vi "2.0.0_Firware Version Check.vi"(6 ".batCM":T1={"Brush_ADC.bat"="Brush_ADC.bat", "Get Release Version.bat"="Get Release Version.bat", "Getting Software  Version.bat"="Getting Software  Version.bat", "Pump_ADC.bat"="Pump_ADC.bat", "Starting  Pump Motor.bat"="Starting  Pump Motor.bat", "Starting  Test Mode.bat"="Starting  Test Mode.bat", "Starting Brush Motor 1.bat"="Starting Brush Motor 1.bat", "Starting Brush Motor 2.bat"="Starting Brush Motor 2.bat", "Starting Brush Motor 3.bat"="Starting Brush Motor 3.bat", "Starting LED Test.bat"="Starting LED Test.bat", "Stopping  Brush Motor.bat"="Stopping  Brush Motor.bat", "Stopping  Pump Motor.bat"="Stopping  Pump Motor.bat", "Stopping  Test Mode.bat"="Stopping  Test Mode.bat", "Starting Self Test.bat"="Starting Self Test.bat", "Software Reset.bat"="Software Reset.bat", "Get HW version.bat"="Get HW version.bat", "Read PMIC status.bat"="Read PMIC status.bat", "SC IMU Data Streaming.bat"="SC IMU Data Streaming.bat"}, 7 "Data in":T2, 8 "error in (no error)":errorcluster, 9 "AllControls In":T3, 10 "?":T4, 11 "Message Queue out":T5) -> (0 "error out":errorcluster, 1 "Flow":string, 2 "Data":T4, 3 "Message Queue Out":T5, 5 "Data out":T2)   [LabVIEW 2017]
uses:
  Depends/AMC/subVIs/TypeDefs/amc_Message Queue.ctl
  Depends/AMC/subVIs/TypeDefs/amc_Message.ctl
  Depends/Tools/Keyed Array/Tools_KeyedArray KeyedArray.ctl
  Ctrls/Data.ctl
  Ctrls/AllControls.ctl
  Ctrls/CSV_Data.ctl
  0516/X682 Chassis Connectivity Tester Program/Ctrls/682_cmd.ctl
types:
  T1 = typedef "682_cmd.ctl" = cluster{"Brush_ADC.bat":string, "Get Release Version.bat":string, "Getting Software  Version.bat":string, "Pump_ADC.bat":string, "Starting  Pump Motor.bat":string, "Starting  Test Mode.bat":string, "Starting Brush Motor 1.bat":string, "Starting Brush Motor 2.bat":string, "Starting Brush Motor 3.bat":string, "Starting LED Test.bat":string, "Stopping  Brush Motor.bat":string, "Stopping  Pump Motor.bat":string, "Stopping  Test Mode.bat":string, "Starting Self Test.bat":string, "Software Reset.bat":string, "Get HW version.bat":string, "Read PMIC status.bat":string, "SC IMU Data Streaming.bat":string}
  T2 = typedef "CSV_Data.ctl" = cluster{"Initialisation":cluster{"LMT - Connect UUT (con COM)":string, "LMT - Software Version (rrel)":string, "LMT - Write SKU file (wskuc)":string, "LMT - SKU file name":string, "Connect UUT DDM":string, "Read DDM EOL Timestamp - Mode":string, "Read DDM EOL Timestamp - Timestamp":string, "Read DDM EOL Timestamp - Rig ID":string, "Read DDM EOL Timestamp - Passmark ID":string, "Read DDM EOL Timestamp - Passmark Rev":string, "Software Version before flashing":string, "Read Hardware Serial":string, "UUT DDM SN":string, "Compare DDM SN with MES SN":string, "Backup PCBA Calibration EEPROM Response - CAL":string, "Flash Firmware Version":string, "Check SW Version":string, "Read DDM SW Version after flashing":string, "Set SKU Config":string, "Ready Status":string, "Set Device Mode to EOL":string, "DDM Parameter - Voltage":string, "DDM Parameter - Current":string, "DDM Parameter - Power":string, "DDM Parameter - Speed":string, "DDM Parameter - Pressure":string, "Tester Parameter - Voltage":string, "Tester Parameter - Current":string, "Tester Parameter - Power":string, "Tester Parameter - Ambient Pressure":string, "Tester Parameter - Ambient Temperature":string, "Calculated Parameter - DDM Pressure Corrected":string, "Calculated Parameter - DDM Real Power":string, "Calculated Parameter - Delta V":string}, "BEMF_Calibration":cluster{"Calibration Result - eol_cold_bemf_temp":string, "DDM Ambient Temp":string, "Restriction Plate Diameter":string, "Calibration Result - eol_bemf_mp_cold_coef_a":string, "Calibration Result - eol_bemf_mp_cold_coef_b":string, "Calibration Result - eol_bemf_mp_cold_coef_c":string, "Calibration Result - eol_bemf_lsi_cold_ref_coeffs":string, "Get - Calibration Result - eol_bemf_lsi_speed":string, "Get - Calibration Result - eol_bemf_lsi_integral_0":string, "Calibration Result - eol_bemf_lsi_integral_1":string, "Get - Calibration Result - eol_bemf_lsi_integral_2":string, "Get - Calibration Result - eol_cold_bemf":string, "Get - Calibration Result - eol_cold_bemf_fisf":string, "Finalise Calibration":string, "Compare -Calibration Result - eol_cold_bemf":string, "Compare -Calibration Result - eol_cold_bemf_fisf":string}, "ECO":cluster{"Reset Power Tune":string, "Reset BEMF FISF Calibration":string, "Restriction Plate Diameter":string, "ECO - Stabilisation Time":string, "ECO - DDM Parameter - Voltage":string, "ECO - DDM Parameter - Current":string, "ECO - DDM Parameter - Power":string, "ECO - DDM Parameter - Measured Power":string, "ECO - DDM Parameter - Speed":string, "ECO - DDM Parameter - Pressure":string, "ECO - Tester Parameter - Voltage":string, "ECO - Tester Parameter - Current":string, "ECO - Tester Parameter - Power":string, "ECO - Tester Parameter - Ambient Pressure":string, "ECO - Tester Parameter - Ambient Temperature":string, "ECO - Tester Parameter - Ambient Humidity":string, "ECO - Calculated Parameter - DDM Pressure Corrected":string, "ECO - Calculated Parameter - DDM Real Power":string, "ECO - Calculated Parameter - Delta V":string, "ECO - Calculated Parameter - Flowrate":string, "ECO - Calculated Parameter - Airwatt":string, "ECO - Formula":string, "PT ECO - Power Tune Mode Status":string}, "BOOST":cluster{"Restriction Plate Diameter":string, "BOOST - Stabilisation Time":string, "BOOST - DDM Parameter - Voltage":string, "BOOST - DDM Parameter - Current":string, "BOOST - DDM Parameter - Power":string, "BOOST - DDM Parameter - Measured Power":string, "BOOST - DDM Parameter - Speed":string, "BOOST - DDM Parameter - Pressure":string, "BOOST - Tester Parameter - Voltage":string, "BOOST - Tester Parameter - Current":string, "BOOST - Tester Parameter - Power":string, "BOOST - Tester Parameter - Ambient Pressure":string, "BOOST - Tester Parameter - Ambient Temperature":string, "BOOST - Tester Parameter - Ambient Humidity":string, "BOOST - Calculated Parameter - DDM Pressure Corrected":string, "BOOST - Calculated Parameter - DDM Real Power":string, "BOOST - Calculated Parameter - Delta V":string, "BOOST - Calculated Parameter - Flowrate":string, "BOOST - Calculated Parameter - Airwatt":string, "BOOST - Get AM Presence":string, "Air Muscle Turn Off Status":string, "BOOST - Air Muscle Calculated Parameter - Airwatt B":string, "BOOST - Air Muscle Calculate Airwatt Delta":string, "PT BOOST - Power Tune Mode Status":string, "Finalise Calibration":string, "ECO - Get AW Calibration value":string, "BOOST - Get AW Calibration value":string}, "MAX":cluster{"Restriction Plate Diameter":string, "MAX - Stabilisation Time":string, "Get Average Delta Tmag (LSIdelta_FISFdelta_LSItmag_FISFtmag_IIRtmag)":string, "Get Average Delta Tmag FISF":string, "MAX - DDM Parameter - Voltage":string, "MAX - DDM Parameter - Current":string, "MAX - DDM Parameter - Power":string, "MAX - DDM Parameter - Measured Power":string, "MAX - DDM Parameter - Speed":string, "MAX - DDM Parameter - Pressure":string, "MAX - Tester Parameter - Voltage":string, "MAX - Tester Parameter - Current":string, "MAX - Tester Parameter - Power":string, "MAX - Tester Parameter - Ambient Pressure":string, "MAX - Tester Parameter - Ambient Temperature":string, "MAX - Tester Parameter - Ambient Humidity":string, "MAX - Calculated Parameter - DDM Pressure Corrected":string, "MAX - Calculated Parameter - DDM Real Power":string, "MAX - Calculated Parameter - Delta V":string, "MAX - Calculated Parameter - Flowrate":string, "MAX - Calculated Parameter - Airwatt":string, "MAX_FISF_Check_Average_Delta_Tmag":string, "MAX - FISF - BEMF Finetune Result":string, "MAX tune - Delta P1":string, "MAX tune - Calculated Parameter - Airwatt":string, "Calculate Delta Airwatts - MAX finetune - Delta P2":string, "MAX finetune - DDM Parameter - Voltage":string, "MAX finetune - DDM Parameter - Current":string, "MAX finetune - DDM Parameter - Power":string, "MAX finetune - DDM Parameter - Measured Power":string, "MAX finetune - DDM Parameter - Speed":string, "MAX finetune - DDM Parameter - Pressure":string, "MAX finetune - Tester Parameter - Voltage":string, "MAX finetune - Tester Parameter - Current":string, "MAX finetune - Tester Parameter - Power":string, "MAX finetune - Tester Parameter - Ambient Pressure":string, "MAX finetune - Tester Parameter - Ambient Temperature":string, "MAX finetune - Tester Parameter - Ambient Humidity":string, "MAX finetune - Calculated Parameter - DDM Pressure Corrected":string, "MAX finetune - Calculated Parameter - DDM Real Power":string, "MAX finetune - Calculated Parameter - Delta V":string, "MAX finetune - Calculated Parameter - Flowrate":string, "MAX finetune - Calculated Parameter - Airwatt":string, "Check Derate Result":string, "Delta Tmag FISF":string, "Get Hot BEMF Result":string, "Calculate delta Pressure":string, "Finalise Calibration":string, "Calculate & Check Delta BEMF":string, "Delta P Airwatts Value":string}, "LL":cluster{"DDM Ambient Temp":string, "Restriction Plate Diameter":string, "LL - DDM Parameter - Voltage":string, "LL - DDM Parameter - Current":string, "LL - DDM Parameter - Power":string, "LL - DDM Parameter - Measured Power":string, "LL - DDM Parameter - Speed":string, "LL - DDM Parameter - Pressure":string, "LL - Tester Parameter - Voltage":string, "LL - Tester Parameter - Current":string, "LL - Tester Parameter - Power":string, "LL - DDM Real Power":string, "LL - Calibrate Task Detect LL":string}, "HL":cluster{"HL - DDM Parameter - Voltage":string, "HL - DDM Parameter - Current":string, "HL - DDM Parameter - Power":string, "HL - DDM Parameter - Measured Power":string, "HL - DDM Parameter - Speed":string, "HL - DDM Parameter - Pressure":string, "HL - Tester Parameter - Voltage":string, "HL - Tester Parameter - Current":string, "HL - Tester Parameter - Power":string, "HL - DDM Real Power":string, "HL - Calibrate Task Detect HL":string}, "LH":cluster{"Restriction Plate Diameter":string, "LH - DDM Parameter - Voltage":string, "LH - DDM Parameter - Current":string, "LH - DDM Parameter - Power":string, "LH - DDM Parameter - Measured Power":string, "LH - DDM Parameter - Speed":string, "LH - DDM Parameter - Pressure":string, "LH - Tester Parameter - Voltage":string, "LH - Tester Parameter - Current":string, "LH - Tester Parameter - Power":string, "LH - DDM Real Power":string, "LH - Calibrate Task Detect LH":string}, "HH":cluster{"HH - DDM Parameter - Voltage":string, "HH - DDM Parameter - Current":string, "HH - DDM Parameter - Power":string, "HH - DDM Parameter - Measured Power":string, "HH - DDM Parameter - Speed":string, "HH - DDM Parameter - Pressure":string, "HH - Tester Parameter - Voltage":string, "HH - Tester Parameter - Current":string, "HH - Tester Parameter - Power":string, "HH - DDM Real Power":string, "HH - Calibrate Task Detect HH":string}, "Inlet Blockage Calibration":cluster{"Inlet Blockage Calibration - DDM Parameter - Voltage":string, "Inlet Blockage Calibration - DDM Parameter - Current":string, "Inlet Blockage Calibration - DDM Parameter - Power":string, "Inlet Blockage Calibration - DDM Parameter - Measured Power":string, "Inlet Blockage Calibration - DDM Parameter - Speed":string, "Inlet Blockage Calibration - DDM Parameter - Pressure":string, "Inlet Blockage Calibration - Tester Parameter - Voltage":string, "Inlet Blockage Calibration - Tester Parameter - Current":string, "Inlet Blockage Calibration - Tester Parameter - Power":string, "Inlet Blockage Calibration - DDM Real Power":string, "Calibration Inlet Blockage_E":string, "Finalise Calibration":string, "Get Task Detect LL":string, "Get Task Detect HL":string, "Get Task Detect LH":string, "Get Task Detect HH":string, "Calibration Inlet Blockage":string, "Calibration eol cold bemf temp":string}, "GOOD":cluster{"GOOD UNIT - Clear EEPROM Error Log":string, "GOOD UNIT - Write Product Timestamp - Mode":string, "GOOD UNIT - Write Product Timestamp - Timestamp":string, "GOOD UNIT - Write Product Timestamp - Rig ID":string, "GOOD UNIT - Write Product Timestamp - Passmark ID":string, "GOOD UNIT - Write Product Timestamp - Passmark Rev":string, "GOOD UNIT - Set Device Mode to PROD":string, "GOOD UNIT - Backup PCBA Calibration EEPROM Response":string, "GOOD UNIT - Check Security Bit":string, "GOOD UNIT - Set Calibration Lock":string, "GOOD UNIT - Get_Calibration_Lock":string, "GOOD UNIT - Disconnect UUT":string}, "NG":cluster{"NG UNIT - Read NVM Error":string, "NG UNIT - Set Device Mode to FCT":string, "NG UNIT - Backup PCBA Calibration EEPROM Response - CAL":string, "NG UNIT - Backup PCBA Calibration EEPROM Response - ERROR":string, "NG UNIT - Backup PCBA Calibration EEPROM Response - USAGE":string, "NG UNIT - Disconnect UUT":string}, "SN":string, "Table":string[][], "Count":cluster{"Total":i32, "OK":i32, "NG":i32, "Yield":dbl}, "Start Time":timestamp, "daemon reference":refnum<k5>, "CT":dbl, "Config":string[][], "OK/NG":bool, "Station ID":string, "MES DDM SN":string, "MES PCBA SN":string, "Retest":string, "Lux":string, "Initialisation_Status":cluster{"LMT - Connect UUT (con COM)":string, "LMT - Software Version (rrel)":string, "LMT - Write SKU file (wskuc)":string, "LMT - SKU file name":string, "Connect UUT DDM":string, "Read DDM EOL Timestamp - Mode":string, "Read DDM EOL Timestamp - Timestamp":string, "Read DDM EOL Timestamp - Rig ID":string, "Read DDM EOL Timestamp - Passmark ID":string, "Read DDM EOL Timestamp - Passmark Rev":string, "Software Version before flashing":string, "Read Hardware Serial":string, "UUT DDM SN":string, "Compare DDM SN with MES SN":string, "Backup PCBA Calibration EEPROM Response - CAL":string, "Flash Firmware Version":string, "Check SW Version":string, "Read DDM SW Version after flashing":string, "Set SKU Config":string, "Ready Status":string, "Set Device Mode to EOL":string, "DDM Parameter - Voltage":string, "DDM Parameter - Current":string, "DDM Parameter - Power":string, "DDM Parameter - Speed":string, "DDM Parameter - Pressure":string, "Tester Parameter - Voltage":string, "Tester Parameter - Current":string, "Tester Parameter - Power":string, "Tester Parameter - Ambient Pressure":string, "Tester Parameter - Ambient Temperature":string, "Calculated Parameter - DDM Pressure Corrected":string, "Calculated Parameter - DDM Real Power":string, "Calculated Parameter - Delta V":string}, "BEMF_Calibration_Status":cluster{"Calibration Result - eol_cold_bemf_temp":string, "DDM Ambient Temp":string, "Restriction Plate Diameter":string, "Calibration Result - eol_bemf_mp_cold_coef_a":string, "Calibration Result - eol_bemf_mp_cold_coef_b":string, "Calibration Result - eol_bemf_mp_cold_coef_c":string, "Calibration Result - eol_bemf_lsi_cold_ref_coeffs":string, "Get - Calibration Result - eol_bemf_lsi_speed":string, "Get - Calibration Result - eol_bemf_lsi_integral_0":string, "Calibration Result - eol_bemf_lsi_integral_1":string, "Get - Calibration Result - eol_bemf_lsi_integral_2":string, "Get - Calibration Result - eol_cold_bemf":string, "Get - Calibration Result - eol_cold_bemf_fisf":string, "Finalise Calibration":string, "Compare -Calibration Result - eol_cold_bemf":string, "Compare -Calibration Result - eol_cold_bemf_fisf":string}, "ECO_Status":cluster{"Reset Power Tune":string, "Reset BEMF FISF Calibration":string, "Restriction Plate Diameter":string, "ECO - Stabilisation Time":string, "ECO - DDM Parameter - Voltage":string, "ECO - DDM Parameter - Current":string, "ECO - DDM Parameter - Power":string, "ECO - DDM Parameter - Measured Power":string, "ECO - DDM Parameter - Speed":string, "ECO - DDM Parameter - Pressure":string, "ECO - Tester Parameter - Voltage":string, "ECO - Tester Parameter - Current":string, "ECO - Tester Parameter - Power":string, "ECO - Tester Parameter - Ambient Pressure":string, "ECO - Tester Parameter - Ambient Temperature":string, "ECO - Tester Parameter - Ambient Humidity":string, "ECO - Calculated Parameter - DDM Pressure Corrected":string, "ECO - Calculated Parameter - DDM Real Power":string, "ECO - Calculated Parameter - Delta V":string, "ECO - Calculated Parameter - Flowrate":string, "ECO - Calculated Parameter - Airwatt":string, "ECO - Formula":string, "PT ECO - Power Tune Mode Status":string}, "BOOST_Status":cluster{"Restriction Plate Diameter":string, "BOOST - Stabilisation Time":string, "BOOST - DDM Parameter - Voltage":string, "BOOST - DDM Parameter - Current":string, "BOOST - DDM Parameter - Power":string, "BOOST - DDM Parameter - Measured Power":string, "BOOST - DDM Parameter - Speed":string, "BOOST - DDM Parameter - Pressure":string, "BOOST - Tester Parameter - Voltage":string, "BOOST - Tester Parameter - Current":string, "BOOST - Tester Parameter - Power":string, "BOOST - Tester Parameter - Ambient Pressure":string, "BOOST - Tester Parameter - Ambient Temperature":string, "BOOST - Tester Parameter - Ambient Humidity":string, "BOOST - Calculated Parameter - DDM Pressure Corrected":string, "BOOST - Calculated Parameter - DDM Real Power":string, "BOOST - Calculated Parameter - Delta V":string, "BOOST - Calculated Parameter - Flowrate":string, "BOOST - Calculated Parameter - Airwatt":string, "BOOST - Get AM Presence":string, "Air Muscle Turn Off Status":string, "BOOST - Air Muscle Calculated Parameter - Airwatt B":string, "BOOST - Air Muscle Calculate Airwatt Delta":string, "PT BOOST - Power Tune Mode Status":string, "Finalise Calibration":string, "ECO - Get AW Calibration value":string, "BOOST - Get AW Calibration value":string}, "MAX_Status":cluster{"Restriction Plate Diameter":string, "MAX - Stabilisation Time":string, "Get Average Delta Tmag (LSIdelta_FISFdelta_LSItmag_FISFtmag_IIRtmag)":string, "Get Average Delta Tmag FISF":string, "MAX - DDM Parameter - Voltage":string, "MAX - DDM Parameter - Current":string, "MAX - DDM Parameter - Power":string, "MAX - DDM Parameter - Measured Power":string, "MAX - DDM Parameter - Speed":string, "MAX - DDM Parameter - Pressure":string, "MAX - Tester Parameter - Voltage":string, "MAX - Tester Parameter - Current":string, "MAX - Tester Parameter - Power":string, "MAX - Tester Parameter - Ambient Pressure":string, "MAX - Tester Parameter - Ambient Temperature":string, "MAX - Tester Parameter - Ambient Humidity":string, "MAX - Calculated Parameter - DDM Pressure Corrected":string, "MAX - Calculated Parameter - DDM Real Power":string, "MAX - Calculated Parameter - Delta V":string, "MAX - Calculated Parameter - Flowrate":string, "MAX - Calculated Parameter - Airwatt":string, "MAX_FISF_Check_Average_Delta_Tmag":string, "MAX - FISF - BEMF Finetune Result":string, "MAX tune - Delta P1":string, "MAX tune - Calculated Parameter - Airwatt":string, "Calculate Delta Airwatts - MAX finetune - Delta P2":string, "MAX finetune - DDM Parameter - Voltage":string, "MAX finetune - DDM Parameter - Current":string, "MAX finetune - DDM Parameter - Power":string, "MAX finetune - DDM Parameter - Measured Power":string, "MAX finetune - DDM Parameter - Speed":string, "MAX finetune - DDM Parameter - Pressure":string, "MAX finetune - Tester Parameter - Voltage":string, "MAX finetune - Tester Parameter - Current":string, "MAX finetune - Tester Parameter - Power":string, "MAX finetune - Tester Parameter - Ambient Pressure":string, "MAX finetune - Tester Parameter - Ambient Temperature":string, "MAX finetune - Tester Parameter - Ambient Humidity":string, "MAX finetune - Calculated Parameter - DDM Pressure Corrected":string, "MAX finetune - Calculated Parameter - DDM Real Power":string, "MAX finetune - Calculated Parameter - Delta V":string, "MAX finetune - Calculated Parameter - Flowrate":string, "MAX finetune - Calculated Parameter - Airwatt":string, "Check Derate Result":string, "Delta Tmag FISF":string, "Get Hot BEMF Result":string, "Calculate delta Pressure":string, "Finalise Calibration":string, "Calculate & Check Delta BEMF":string, "Delta P Airwatts Value":string}, "LL_Status":cluster{"DDM Ambient Temp":string, "Restriction Plate Diameter":string, "LL - DDM Parameter - Voltage":string, "LL - DDM Parameter - Current":string, "LL - DDM Parameter - Power":string, "LL - DDM Parameter - Measured Power":string, "LL - DDM Parameter - Speed":string, "LL - DDM Parameter - Pressure":string, "LL - Tester Parameter - Voltage":string, "LL - Tester Parameter - Current":string, "LL - Tester Parameter - Power":string, "LL - DDM Real Power":string, "LL - Calibrate Task Detect LL":string}, "HL_Status":cluster{"HL - DDM Parameter - Voltage":string, "HL - DDM Parameter - Current":string, "HL - DDM Parameter - Power":string, "HL - DDM Parameter - Measured Power":string, "HL - DDM Parameter - Speed":string, "HL - DDM Parameter - Pressure":string, "HL - Tester Parameter - Voltage":string, "HL - Tester Parameter - Current":string, "HL - Tester Parameter - Power":string, "HL - DDM Real Power":string, "HL - Calibrate Task Detect HL":string}, "LH_Status":cluster{"Restriction Plate Diameter":string, "LH - DDM Parameter - Voltage":string, "LH - DDM Parameter - Current":string, "LH - DDM Parameter - Power":string, "LH - DDM Parameter - Measured Power":string, "LH - DDM Parameter - Speed":string, "LH - DDM Parameter - Pressure":string, "LH - Tester Parameter - Voltage":string, "LH - Tester Parameter - Current":string, "LH - Tester Parameter - Power":string, "LH - DDM Real Power":string, "LH - Calibrate Task Detect LH":string}, "HH_Status":cluster{"HH - DDM Parameter - Voltage":string, "HH - DDM Parameter - Current":string, "HH - DDM Parameter - Power":string, "HH - DDM Parameter - Measured Power":string, "HH - DDM Parameter - Speed":string, "HH - DDM Parameter - Pressure":string, "HH - Tester Parameter - Voltage":string, "HH - Tester Parameter - Current":string, "HH - Tester Parameter - Power":string, "HH - DDM Real Power":string, "HH - Calibrate Task Detect HH":string}, "Inlet Blockage Calibration_Status":cluster{"Inlet Blockage Calibration - DDM Parameter - Voltage":string, "Inlet Blockage Calibration - DDM Parameter - Current":string, "Inlet Blockage Calibration - DDM Parameter - Power":string, "Inlet Blockage Calibration - DDM Parameter - Measured Power":string, "Inlet Blockage Calibration - DDM Parameter - Speed":string, "Inlet Blockage Calibration - DDM Parameter - Pressure":string, "Inlet Blockage Calibration - Tester Parameter - Voltage":string, "Inlet Blockage Calibration - Tester Parameter - Current":string, "Inlet Blockage Calibration - Tester Parameter - Power":string, "Inlet Blockage Calibration - DDM Real Power":string, "Calibration Inlet Blockage_E":string, "Finalise Calibration":string, "Get Task Detect LL":string, "Get Task Detect HL":string, "Get Task Detect LH":string, "Get Task Detect HH":string, "Calibration Inlet Blockage":string, "Calibration eol cold bemf temp":string}, "GOOD_Status":cluster{"GOOD UNIT - Clear EEPROM Error Log":string, "GOOD UNIT - Write Product Timestamp - Mode":string, "GOOD UNIT - Write Product Timestamp - Timestamp":string, "GOOD UNIT - Write Product Timestamp - Rig ID":string, "GOOD UNIT - Write Product Timestamp - Passmark ID":string, "GOOD UNIT - Write Product Timestamp - Passmark Rev":string, "GOOD UNIT - Set Device Mode to PROD":string, "GOOD UNIT - Backup PCBA Calibration EEPROM Response":string, "GOOD UNIT - Check Security Bit":string, "GOOD UNIT - Set Calibration Lock":string, "GOOD UNIT - Get_Calibration_Lock":string, "GOOD UNIT - Disconnect UUT":string}, "NG_Status":cluster{"NG UNIT - Read NVM Error":string, "NG UNIT - Set Device Mode to FCT":string, "NG UNIT - Backup PCBA Calibration EEPROM Response - CAL":string, "NG UNIT - Backup PCBA Calibration EEPROM Response - ERROR":string, "NG UNIT - Backup PCBA Calibration EEPROM Response - USAGE":string, "NG UNIT - Disconnect UUT":string}, "SKU":string, "Plate_Diameter":string, "Alarm":string}
  T3 = typedef "AllControls.ctl" = cluster{"MainVI":refnum<vi>, "AlarmInfo":refnum<vi>, "Log":refnum<vi>, "Current CT":refnum<vi>, "ProductID":refnum<vi>, "Device state":refnum<vi>, "MES":refnum<vi>, "mode":refnum<vi>, "TestInfo":refnum<vi>, "SubPnl":refnum<vi>, "Table":refnum<vi>, "MES bool":refnum<vi>, "TestMode":refnum<vi>, "Recipe":refnum<vi>, "Fail resume":refnum<vi>, "LogIn":refnum<vi>, "Start":refnum<vi>, "Maintenance":refnum<vi>, "Stop":refnum<vi>, "Exit":refnum<vi>}
  T4 = typedef "Data.ctl" = cluster{"Initialisation":cluster{"DDM_Parameter":dbl[], "DDM_Parameter_status":bool[], "Get_Tester_Parameter":dbl[], "Get_Tester_Parameter_status":bool[], "Cal_Tester_Parameter":dbl[], "Cal_Tester_Parameter_status":bool[], "sw_version_before_status":bool, "sw_version_after_status":bool, "Set_SKU_Config_With_LMT_status":bool, "FCT_timestamp_status":bool, "LMT_Connect_to_UUT_status":bool}, "BEMF_Calibration":cluster{"Read_ambient_temperature":dbl, "Calibration_Vaule":dbl[], "Calibration_Vaule _B":dbl[], "Calibration_Vaule_status":bool[], "Calibration_Vaule_B_status":bool[]}, "ECO":cluster{"DDM_Parameter":dbl[], "DDM_Parameter_status":bool[], "Get_Tester_Parameter":dbl[], "Get_Tester_Parameter_status":bool[], "Cal_Tester_Parameter":dbl[], "Cal_Tester_Parameter_status":bool[], "DDM_Parameter_after_power_tune":dbl[], "Get_Tester_Parameter_after_power_tune":dbl[], "Cal_Tester_Parameter_after_power_tune":dbl[], "Cal_Tester_Parameter_after_power_tune_status":bool[], "Delta_P":dbl}, "BOOST":cluster{"DDM_Parameter":dbl[], "DDM_Parameter_status":bool[], "Get_Tester_Parameter":dbl[], "Get_Tester_Parameter_status":bool[], "Cal_Tester_Parameter":dbl[], "Cal_Tester_Parameter_status":bool[], "DDM_Parameter_after_power_tune":dbl[], "Get_Tester_Parameter_after_power_tune":dbl[], "Cal_Tester_Parameter_after_power_tune":dbl[], "Cal_Tester_Parameter_after_power_tune_status":bool[], "airwatts_am_off":dbl, "AW_Delta_(AM_on_and_off)":dbl, "AW_Delta_(AM_on_and_off)_Status":bool, "Delta_P":dbl}, "MAX":cluster{"Average_Tmag_Data":cluster{"LSI Delta in degC":dbl, "FISF Delta in degc":dbl, "LSI Tmag in degC":dbl, "Fisf Tmag in degC":dbl, "IIR Tmag in degC":dbl}, "DDM_Parameter":dbl[], "DDM_Parameter_status":bool[], "Get_Tester_Parameter":dbl[], "Get_Tester_Parameter_status":bool[], "Cal_Tester_Parameter":dbl[], "BEMF_Finetune":cluster{"eol_bemf_mp_cold_coef_c":dbl, "eol_cold_bemf_fisf_offset":dbl}, "AW_Tune":cluster{"delta_P1":dbl, "delta_P_Setting":dbl}, "DDM_Parameter_after_Airwatts_Tune":dbl[], "Get_Tester_Parameter_after_Airwatts_Tune":dbl[], "Cal_Tester_Parameter_after_Airwatts_Tune":dbl[], "DDM_Parameter_after_Airwatts_Finetune":dbl[], "Get_Tester_Parameter_after_Airwatts_Finetune":dbl[], "Cal_Tester_Parameter_after_Airwatts_Finetune":dbl[], "AW_Finetune":cluster{"delta_P2":dbl, "delta_P_Setting":dbl}, "Delta_Tmag_after_tune":cluster{"LSI Delta in degC":dbl, "FISF Delta in degc":dbl, "LSI Tmag in degC":dbl, "Fisf Tmag in degC":dbl, "IIR Tmag in degC":dbl}, "Hot Bemf in mV":dbl, "DDM_Pressure":dbl, "Delta_Pressure":dbl, " Cold Bemf in mV":dbl, " delta Bemf":dbl, " delta p":dbl, "Delta_Pressure_status":bool, " delta Bemf_status":bool, "LSI Delta in degC_status":bool, "FISF Delta in degc_status":bool, "Max_check_derate_status_status":bool, "Average_All_data":dbl[][], "Average_Tmag_Data_status":bool[], "Average_Tmag_Data_after_tune_status":bool[], "Cal_Tester_Parameter_status":bool[], "Cal_Tester_Parameter_status_after_Airwatts_Tune":bool[], "Cal_Tester_Parameter_status_after_Airwatts_FineTune":bool[]}, "Task_Detect_Calib":cluster{"LL":cluster{"DDM_Parameter":dbl[], "DDM_Parameter_status":bool[], "Get_Tester_Parameter":dbl[], "Get_Tester_Parameter_status":bool[], "Set_task_detect_A":dbl, "Set_task_detect_A_Status":bool}, "HL":cluster{"DDM_Parameter":dbl[], "DDM_Parameter_status":bool[], "Get_Tester_Parameter":dbl[], "Get_Tester_Parameter_status":bool[], "Set_task_detect_B":dbl, "Set_task_detect_B_Status":bool}, "LH":cluster{"DDM_Parameter":dbl[], "DDM_Parameter_status":bool[], "Get_Tester_Parameter":dbl[], "Get_Tester_Parameter_status":bool[], "Set_task_detect_C":dbl, "Set_task_detect_C_Status":bool}, "HH":cluster{"DDM_Parameter":dbl[], "DDM_Parameter_status":bool[], "Get_Tester_Parameter":dbl[], "Get_Tester_Parameter_status":bool[], "Set_task_detect_D":dbl, "Read_and_check_calibration_Status":bool[], "Set_task_detect_D_Status":bool}, "Get_eol_inlet_blockage_E":dbl, "Calib_vaule":cluster{"Get_task_detect_LL":dbl, "Get_task_detect_HL":dbl, "Get_task_detect_LH":dbl, "Get_task_detect_HH":dbl, "eol_inlet_blockage":dbl, "eol_code_bemf_temp":dbl}, "calibrated temp":dbl, "Inlet_Blockage_Calibration":cluster{"DDM_Parameter":dbl[], "DDM_Parameter_status":bool[], "Get_Tester_Parameter":dbl[], "Get_Tester_Parameter_status":bool[]}, "Get_eol_inlet_blockage_E_Status":bool}, "good":cluster{"Write_Product_TS":cluster{"TIMESTAMP":i64, "RIG_ID":i64, "PASSMARK_ID":i64, "PASSMARK_REV":i64}, "Read_Product_TS":cluster{"TIMESTAMP":i64, "RIG_ID":i64, "PASSMARK_ID":i64, "PASSMARK_REV":i64}, "Good_Check_Secuity_Bit_Stauts":bool}}
  T5 = typedef "amc_Message Queue.ctl" = refnum<queue>
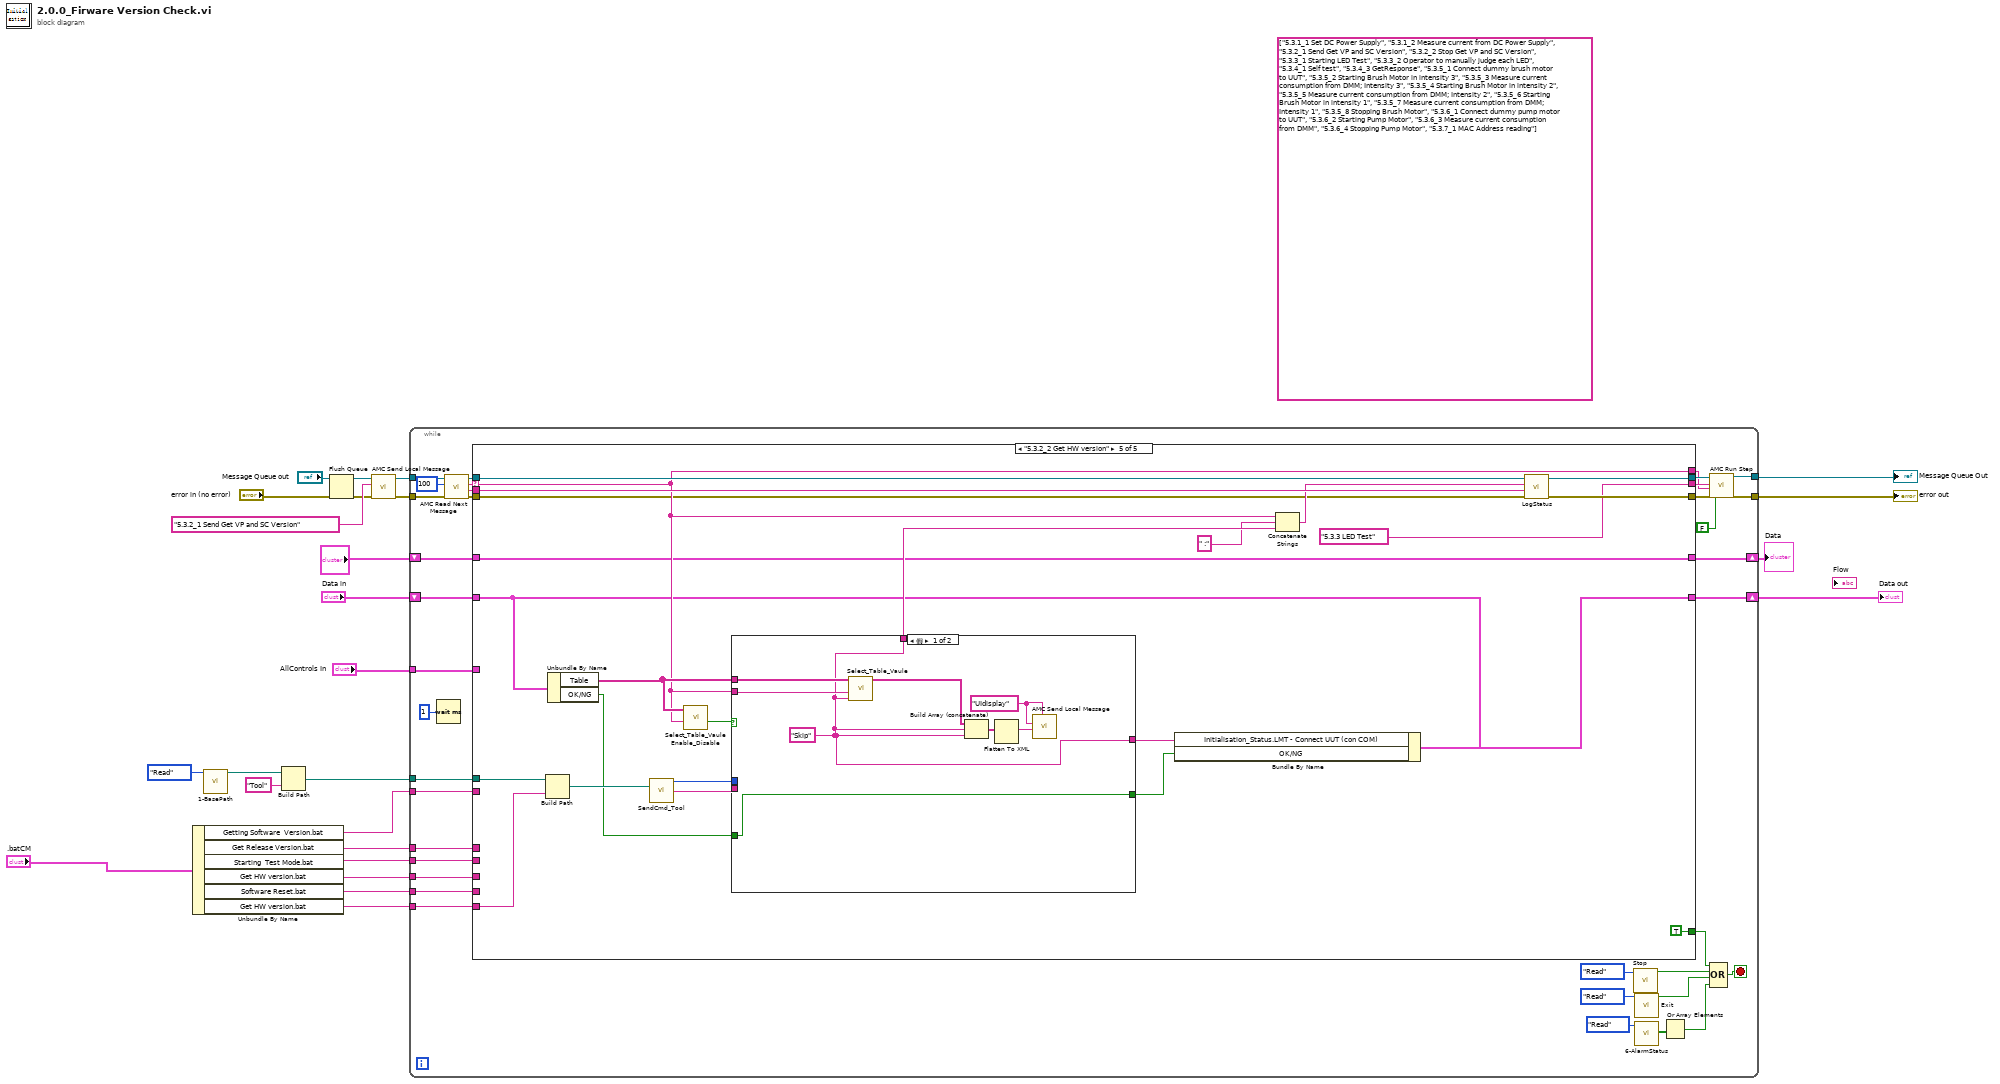
[diagram p0: block diagram]
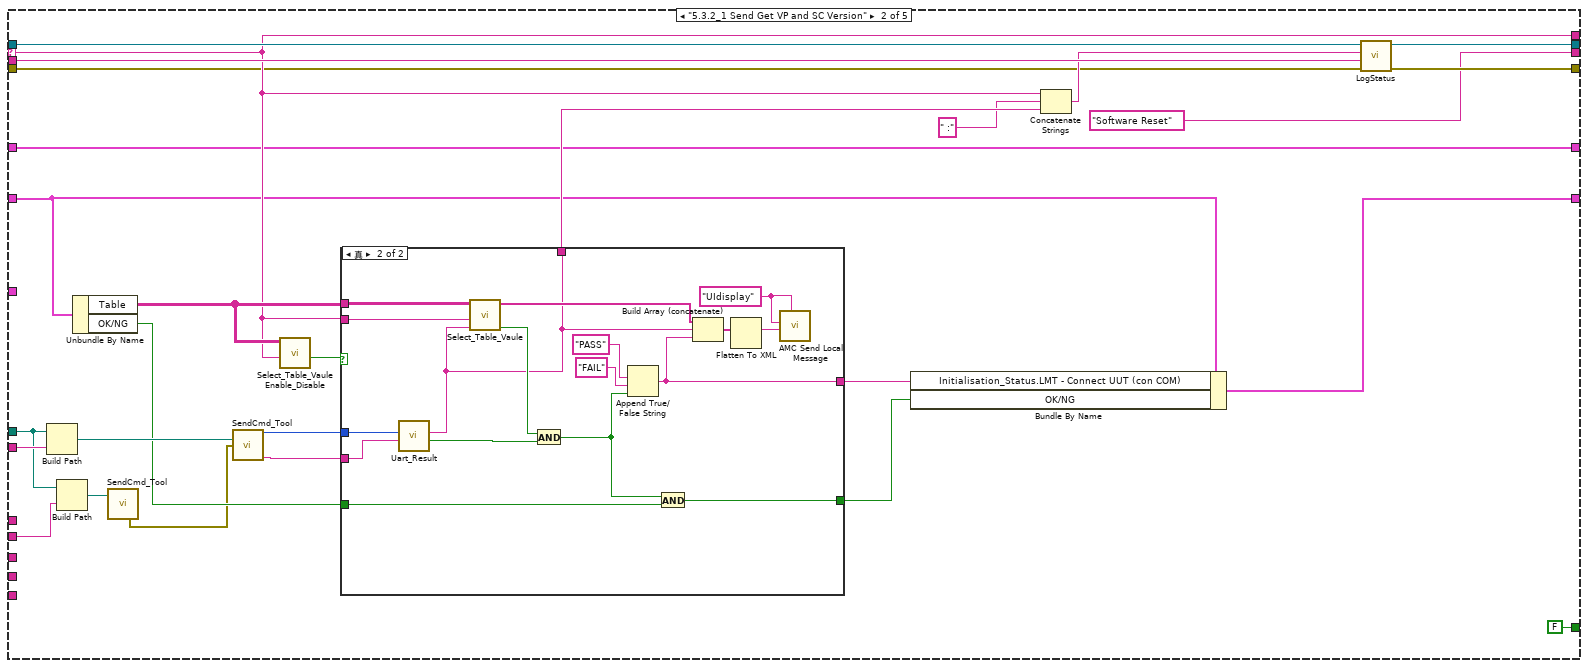
[diagram p3: hidden frame]
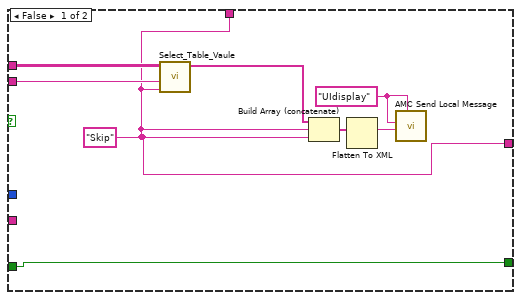
[diagram p4: hidden frame]
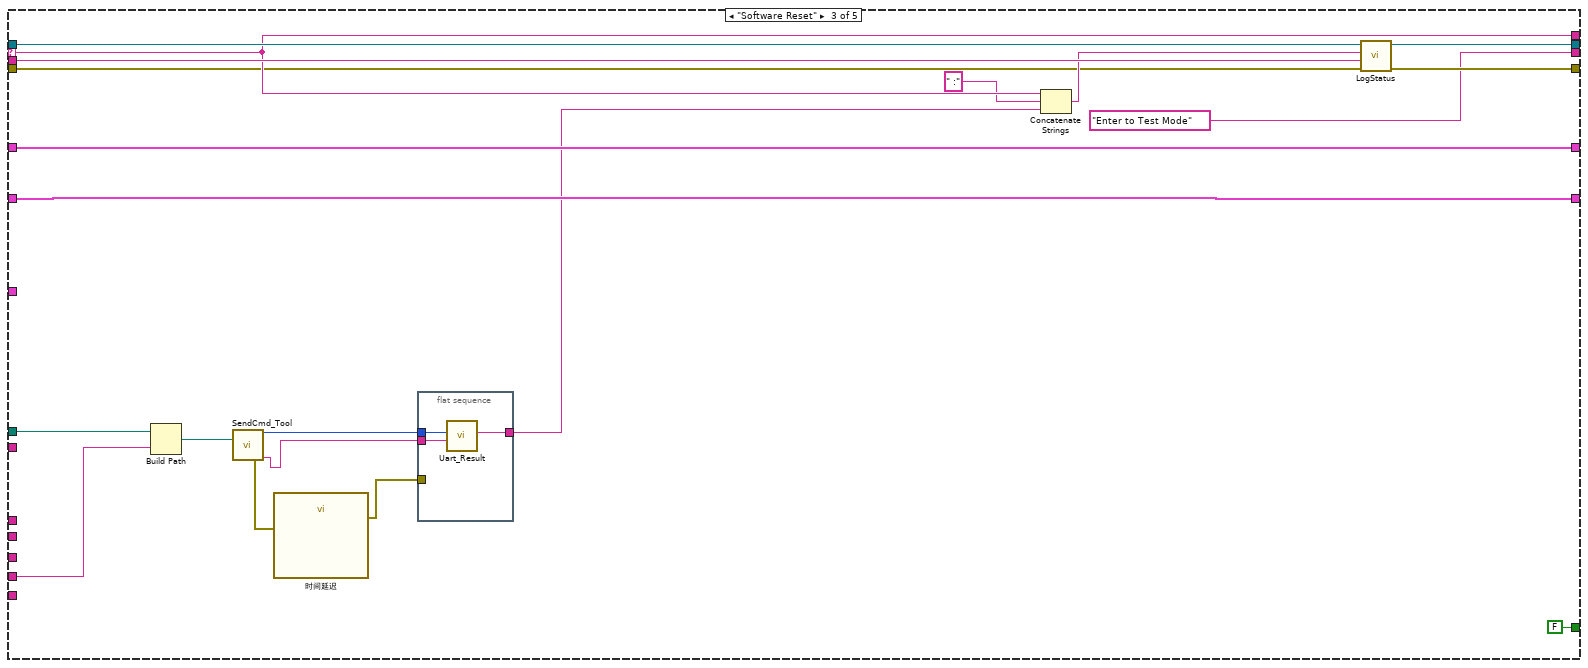
[diagram p5: hidden frame]
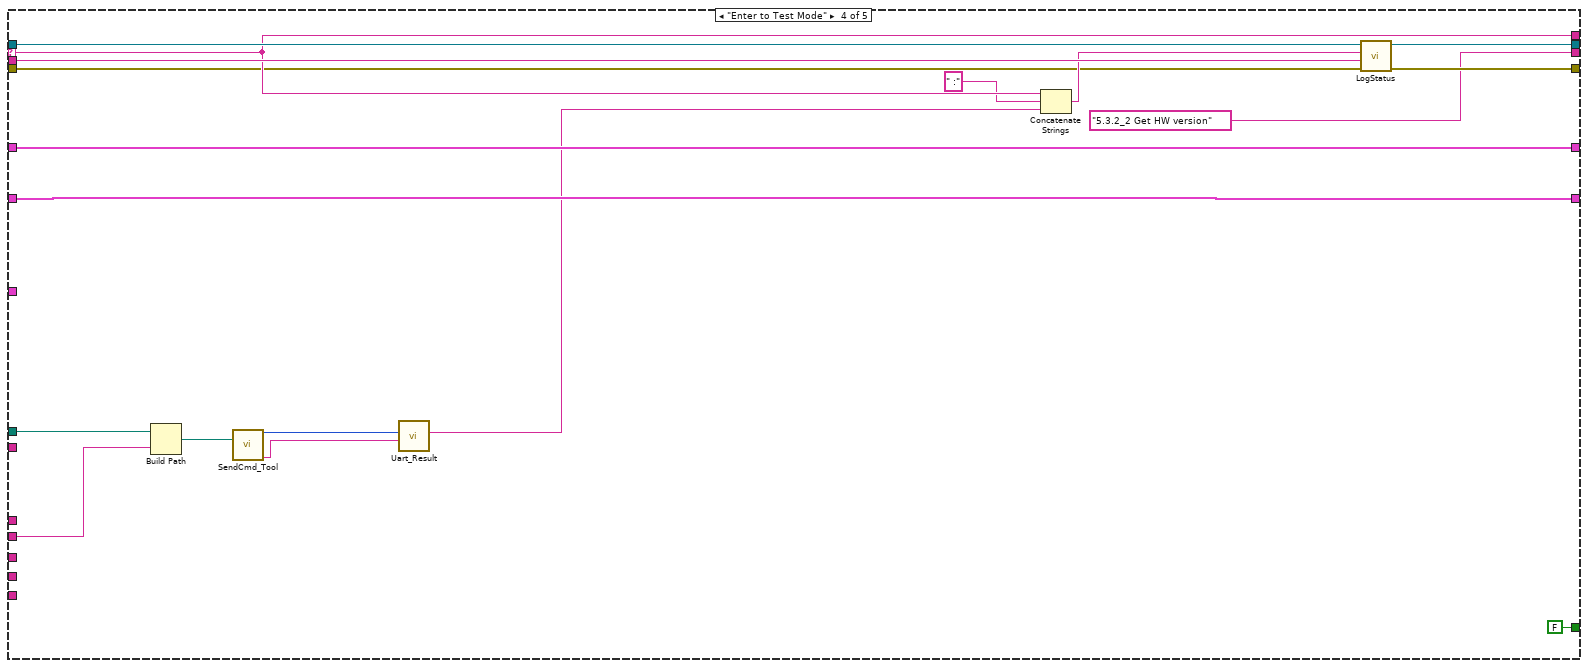
[diagram p6: hidden frame]
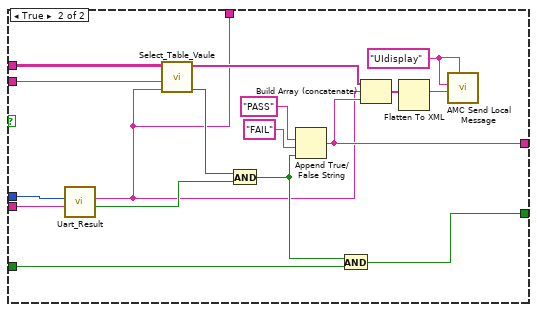
[diagram p7: hidden frame]
diagram:
  (unwired) string[] ["5.3.1_1 Set DC Power Supply", "5.3.1_2 Measure current from DC Power Supply", "5.3.2_1 Send Get VP and SC Version", "5.3.2_2 Stop Get VP and SC Version", "5.3.3_1 Starting LED Test", "5.3.3_2 Operator to manually judge each LED", "5.3.4_1 Self test", "5.3.4_3 GetResponse", "5.3.5_1 Connect dummy brush motor to UUT", "5.3.5_2 Starting Brush Motor in intensity 3", "5.3.5_3 Measure current consumption from DMM; Intensity 3", "5.3.5_4 Starting Brush Motor in intensity 2", "5.3.5_5 Measure current consumption from DMM; Intensity 2", "5.3.5_6 Starting Brush Motor in intensity 1", "5.3.5_7 Measure current consumption from DMM; Intensity 1", "5.3.5_8 Stopping Brush Motor", "5.3.6_1 Connect dummy pump motor to UUT", "5.3.6_2 Starting Pump Motor", "5.3.6_3 Measure current consumption from DMM", "5.3.6_4 Stopping Pump Motor", "5.3.7_1 MAC Address reading"] ("subarray")
  n1 = Unbundle By Name(".batCM") -> ("Getting Software  Version.bat"=w7:string, "Get Release Version.bat"=w6:string, "Starting  Test Mode.bat"=w5:string, "Get HW version.bat"=w3:string, "Software Reset.bat"=w2:string, "Get HW version.bat"=w1:string)
  n2 = call "1-BasePath.vi"("Step"=enum16{"Initial", "Write", "Read"}."Read") -> ("Path Out"=w9:path)  [unwired: 9 in, 1 out]
  n3 = Build Path(base path=w9, name or relative path="Tool") -> (appended path=w8:path)
  n4 = Flush Queue(queue="Message Queue out") -> (queue out=w17:T5)  [unwired: 1 in, 2 out]
  n5 = call "AMC Send Local Message.vi"("error in (no error)"="error in (no error)", "Message Name"="5.3.2_1 Send Get VP and SC Version", "Message Queue in"=w17) -> ("error out"=w21:errorcluster, "Message Queue out"=w22:T5)  [unwired: 7 in]
  n6 = while {
    tunnel: w22 -> [w60]
    tunnel: [w56] -> w16
    tunnel: w21 -> [w54]
    tunnel: [w51] -> w15
    shift-right: [w47] -> w18
    shift-left: "?" -> [w48]
    tunnel: "AllControls In" -> [w37]
    shift-right: [w35] -> w12
    shift-left: "Data in" -> [w36]
    tunnel: w8 -> [w31]
    tunnel: w7 -> [w30]
    tunnel: w6 -> [w29]
    tunnel: w5 -> [w28]
    tunnel: w3 -> [w27]
    tunnel: w2 -> [w26]
    tunnel: w1 -> [w25]
    stop <- w40 stop-if-true
    n7 = Wait (ms)(milliseconds to wait=u32 1 ("等待时间（毫秒）")) -> ()  [unwired: 1 out]
    n8 = call "AMC Read Next Message.vi"("error in (no error)"=w54, "timeout (1ms)"=100, "Message Queue in"=w60) -> ("error out"=w53:errorcluster, "Message Value"=w45:string, "Message Name"=w58:string, "Message Queue out"=w59:T5)  [unwired: 1 in, 4 out]
    n9 = case shown="\"5.3.2_2 Get HW version\"" w58 {
      selector: w58 -> [_ w85 w130 w150 w172]
      tunnel: w59 -> [w64 w90 w134 w154 w177]
      tunnel: [w64 w90 w134 w154 w177] -> w57
      tunnel: w53 -> [w63 w84 w129 w149 w171]
      tunnel: [w63 w89 w133 w153 w176] -> w52
      tunnel: [_ FALSE ("GRR") FALSE ("GRR") FALSE ("GRR") TRUE ("GRR")] -> w41
      tunnel: w48 -> [w62 w80 w127 w147 w167]
      tunnel: [w62 w80 w127 w147 w167] -> w47
      tunnel: w45 -> [_ w88 w132 w152 w175]
      tunnel: [_ w85 w130 w150 w172] -> w44
      tunnel: [_ "Software Reset" "Enter to Test Mode" "5.3.2_2 Get HW version" "5.3.3 LED Test"] -> w46
      tunnel: w37 -> [_ _ _ _ _]
      tunnel: w36 -> [w61 w79 w120 w141 w166]
      tunnel: [w61 w78 w120 w141 w165] -> w35
      tunnel: w31 -> [_ w67 w121 w142 w161]
      tunnel: w30 -> [_ w72 _ _ _]
      tunnel: w29 -> [_ _ _ _ _]
      tunnel: w28 -> [_ w66 _ w139 _]
      tunnel: w27 -> [_ _ _ _ _]
      tunnel: w26 -> [_ _ w119 _ _]
      tunnel: w25 -> [_ _ _ _ w155]
      frame "假", Default {
      }
      frame "5.3.2_1 Send Get VP and SC Version" {
        n10 = Build Path(base path=w67, name or relative path=w72) -> (appended path=w71:path)
        n11 = Build Path(base path=w67, name or relative path=w66) -> (appended path=w68:path)
        n12 = Unbundle By Name(w79) -> ("Table"=w86:string[][], "OK/NG"=w70:bool)
        n13 = call "SendCmd_Tool.vi"("path_bat"=w68) -> ("error out 3"=w65:errorcluster)  [unwired: 6 in, 8 out]
        n14 = call "SendCmd_Tool.vi"("path_bat"=w71, "error in (no error) 2"=w65) -> ("return code"=w74:i32, "version info"=w75:string)  [unwired: 5 in, 7 out]
        n15 = call "Select_Table_Vaule Enable_Disable.vi"("Action"=w85, "Table"=w86) -> ("Enable"=w82:bool)  [unwired: 8 in, 1 out]
        n16 = case shown="真" w82 {
          tunnel: [w92 w99] -> w83
          tunnel: w86 -> [w94 w109]
          tunnel: w85 -> [w93 w108]
          tunnel: w75 -> [_ w101]
          tunnel: [w92 w107] -> w77
          tunnel: w74 -> [_ w102]
          tunnel: [w91 w103] -> w73
          tunnel: w70 -> [w91 w104]
          frame False {
            w98 = "UIdisplay" ("Process (\"\" - local)")
            w92 = "Skip" ("Action")
            n17 = call "Select_Table_Vaule.vi"("Vaule"=w92, "Action"=w93, "Table"=w94) -> ("vaule"=w95:string[])  [unwired: 7 in, 1 out]
            n18 = Build Array (concatenate)(w95, w92, w92) -> (w97:string[])
            n19 = Flatten To XML(anything=w97) -> (xml string=w96:string)
            n20 = call "AMC Send Local Message.vi"("Process (\"\" - local)"=w98, "Message Value"=w96, "Message Name"=w98) -> ()  [unwired: 7 in, 2 out]
          }
          frame True {
            w114 = "UIdisplay" ("Process (\"\" - local)")
            n21 = call "Uart_Result.vi"("input"=w101, "return code"=w102) -> ("Command Sucess"=w100:bool, "return_result"=w99:string)  [unwired: 8 in]
            n22 = call "Select_Table_Vaule.vi"("Vaule"=w99, "Action"=w108, "Table"=w109) -> ("Result"=w106:bool, "vaule"=w115:string[])  [unwired: 7 in]
            n23 = And(x=w106, y=w100) -> (x .and. y?=w105:bool)
            n24 = Append True/False String(1:w105, 2:"FAIL" ("真字符串"), 3:"PASS" ("真字符串")) -> (0:w107:string)  [unwired: 1 in]
            n25 = And(x=w105, y=w104) -> (x .and. y?=w103:bool)
            n26 = Build Array (concatenate)(w115, w99, w107) -> (w113:string[])
            n27 = Flatten To XML(anything=w113) -> (xml string=w112:string)
            n28 = call "AMC Send Local Message.vi"("Process (\"\" - local)"=w114, "Message Value"=w112, "Message Name"=w114) -> ()  [unwired: 7 in, 2 out]
          }
        }
        n29 = Bundle By Name(cluster=w79, "Initialisation_Status.LMT - Connect UUT (con COM)"=w77, "OK/NG"=w73) -> (w78:T2)
        n30 = Concatenate Strings(w85, " :", w83) -> (w87:string)
        n31 = call "LogStatus.vi"("error in (no error)"=w84, "last message"=w88, "message"=w87) -> ("error  out"=w89:errorcluster)  [unwired: 8 in]
      }
      frame "Software Reset" {
        n32 = Build Path(base path=w121, name or relative path=w119) -> (appended path=w123:path)
        n33 = call "SendCmd_Tool.vi"("path_bat"=w123) -> ("return code"=w124:i32, "error out 3"=w117:errorcluster, "version info"=w125:string)  [unwired: 6 in, 6 out]
        n34 = call "时间延迟"("error in (no error)"=w117) -> ("error out"=w116:errorcluster)  [unwired: 10 in]
        n35 = flat-sequence {
          tunnel: w125 -> [w137]
          tunnel: w124 -> [w136]
          tunnel: [w135] -> w118
          tunnel: w116 -> [_]
          frame #0 {
            n36 = call "Uart_Result.vi"("input"=w137, "return code"=w136) -> ("return_result"=w135:string)  [unwired: 8 in, 1 out]
          }
        }
        n37 = Concatenate Strings(w130, " :", w118) -> (w131:string)
        n38 = call "LogStatus.vi"("error in (no error)"=w129, "last message"=w132, "message"=w131) -> ("error  out"=w133:errorcluster)  [unwired: 8 in]
      }
      frame "Enter to Test Mode" {
        n39 = Build Path(base path=w142, name or relative path=w139) -> (appended path=w144:path)
        n40 = call "SendCmd_Tool.vi"("path_bat"=w144) -> ("return code"=w145:i32, "version info"=w138:string)  [unwired: 6 in, 7 out]
        n41 = call "Uart_Result.vi"("input"=w138, "return code"=w145) -> ("return_result"=w140:string)  [unwired: 8 in, 1 out]
        n42 = Concatenate Strings(w150, " :", w140) -> (w151:string)
        n43 = call "LogStatus.vi"("error in (no error)"=w149, "last message"=w152, "message"=w151) -> ("error  out"=w153:errorcluster)  [unwired: 8 in]
      }
      frame "5.3.2_2 Get HW version" {
        n44 = Build Path(base path=w161, name or relative path=w155) -> (appended path=w160:path)
        n45 = Unbundle By Name(w166) -> ("Table"=w173:string[][], "OK/NG"=w159:bool)
        n46 = call "SendCmd_Tool.vi"("path_bat"=w160) -> ("return code"=w158:i32, "release version:"=w157:string)  [unwired: 6 in, 7 out]
        n47 = call "Select_Table_Vaule Enable_Disable.vi"("Action"=w172, "Table"=w173) -> ("Enable"=w169:bool)  [unwired: 8 in, 1 out]
        n48 = case shown="假" w169 {
          tunnel: [w179 w186] -> w170
          tunnel: w173 -> [w181 w196]
          tunnel: w172 -> [w180 w195]
          tunnel: [w179 w194] -> w164
          tunnel: [w178 w190] -> w162
          tunnel: w159 -> [w178 w191]
          tunnel: w158 -> [_ w189]
          tunnel: w157 -> [_ w188]
          frame False {
            w185 = "UIdisplay" ("Process (\"\" - local)")
            w179 = "Skip" ("Action")
            n49 = call "Select_Table_Vaule.vi"("Vaule"=w179, "Action"=w180, "Table"=w181) -> ("vaule"=w182:string[])  [unwired: 7 in, 1 out]
            n50 = Build Array (concatenate)(w182, w179, w179) -> (w184:string[])
            n51 = Flatten To XML(anything=w184) -> (xml string=w183:string)
            n52 = call "AMC Send Local Message.vi"("Process (\"\" - local)"=w185, "Message Value"=w183, "Message Name"=w185) -> ()  [unwired: 7 in, 2 out]
          }
          frame True {
            w201 = "UIdisplay" ("Process (\"\" - local)")
            n53 = call "Uart_Result.vi"("input"=w188, "return code"=w189) -> ("Command Sucess"=w187:bool, "return_result"=w186:string)  [unwired: 8 in]
            n54 = call "Select_Table_Vaule.vi"("Vaule"=w186, "Action"=w195, "Table"=w196) -> ("Result"=w193:bool, "vaule"=w202:string[])  [unwired: 7 in]
            n55 = And(x=w193, y=w187) -> (x .and. y?=w192:bool)
            n56 = Append True/False String(1:w192, 2:"FAIL" ("真字符串"), 3:"PASS" ("真字符串")) -> (0:w194:string)  [unwired: 1 in]
            n57 = And(x=w192, y=w191) -> (x .and. y?=w190:bool)
            n58 = Build Array (concatenate)(w202, w186, w194) -> (w200:string[])
            n59 = Flatten To XML(anything=w200) -> (xml string=w199:string)
            n60 = call "AMC Send Local Message.vi"("Process (\"\" - local)"=w201, "Message Value"=w199, "Message Name"=w201) -> ()  [unwired: 7 in, 2 out]
          }
        }
        n61 = Bundle By Name(cluster=w166, "Initialisation_Status.LMT - Connect UUT (con COM)"=w164, "OK/NG"=w162) -> (w165:T2)
        n62 = Concatenate Strings(w172, " :", w170) -> (w174:string)
        n63 = call "LogStatus.vi"("error in (no error)"=w171, "last message"=w175, "message"=w174) -> ("error  out"=w176:errorcluster)  [unwired: 8 in]
      }
    }
    n64 = call "Stop.vi"("Step"=enum16{"Initial", "Write", "Read"}."Read") -> ("Stop Out"=w39:bool)  [unwired: 9 in, 1 out]
    n65 = call "Exit.vi"("Step"=enum16{"Initial", "Write", "Read"}."Read" ("step")) -> ("Exit Out"=w38:bool)  [unwired: 9 in, 1 out]
    n66 = call "6-AlarmStatus.vi"("Step"=enum16{"Initial", "Write", "Read"}."Read") -> ("AlarmValue Out"=w33:bool[])  [unwired: 9 in, 1 out]
    n67 = Or Array Elements(Boolean array=w33) -> (logical OR=w32:bool)
    n68 = call "AMC Run Step.vi"("Message Queue In"=w57, "Message Name"=w46, "Message Value"=w44, "error in (no error)"=w52, "Mli/Sig"=FALSE) -> ("Message Queue Out"=w56:T5, "error out"=w51:errorcluster)  [unwired: 13 in]
    n69 = Compound Arithmetic op=OR(w41, w39, w38, w32) -> (w40:bool)
  }
  "Message Queue Out" <- w16
  "error out" <- w15
  "Data" <- w18
  "Data out" <- w12
